vi "S2C_OM8257_Proc_Commands.vi"(7 "VI_Ref":refnum<vi>, 8 "Error In":errorcluster, 10 "Settings":T1, 11 "Q-Ref":refnum<queue>) -> (0 "Error Out":errorcluster, 2 "Stop?":bool, 3 "Response":variant)   [LabVIEW 2015]
uses:
  S2C_OM8257_Proc_Globals.vi
  _Shared/S2C_Shared_Proc_Globals.vi
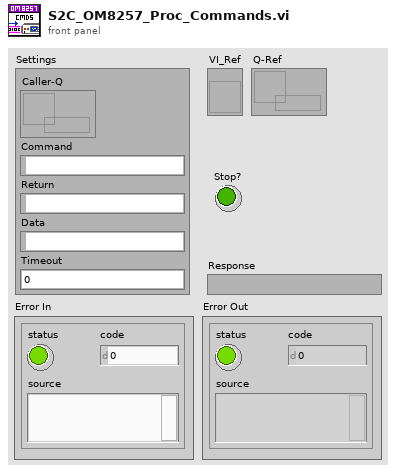
[diagram p1: front panel]
types:
  T1 = cluster{"Caller-Q":refnum<queue>, "Command":string, "Return":string, "Data":variant, "Timeout":dbl}
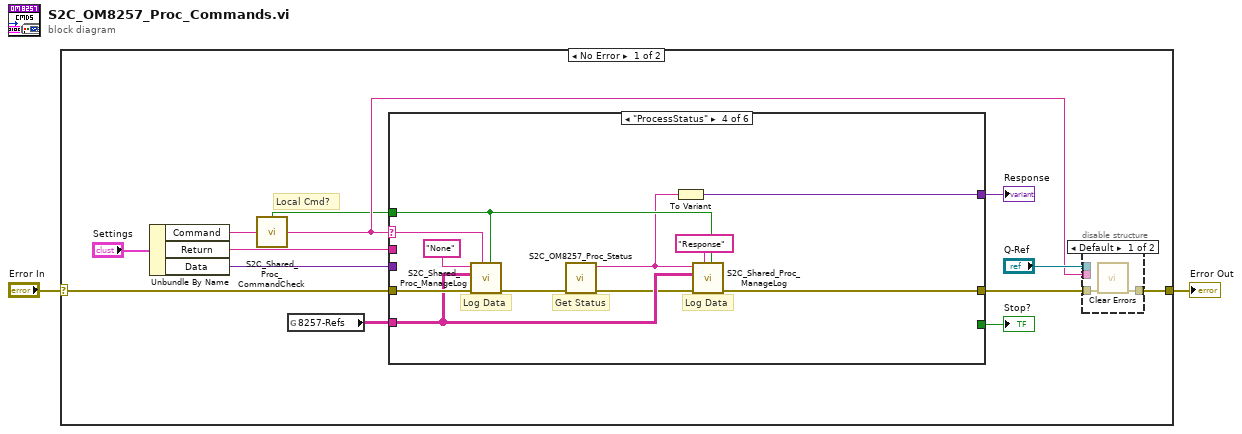
[diagram p0: block diagram]
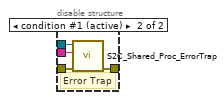
[diagram p2: hidden frame]
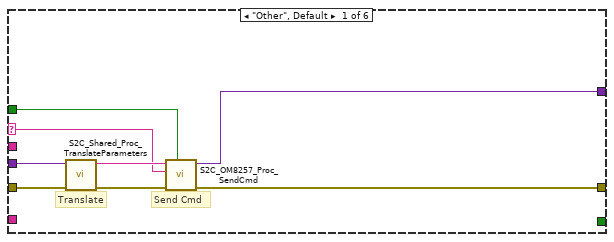
[diagram p3: hidden frame]
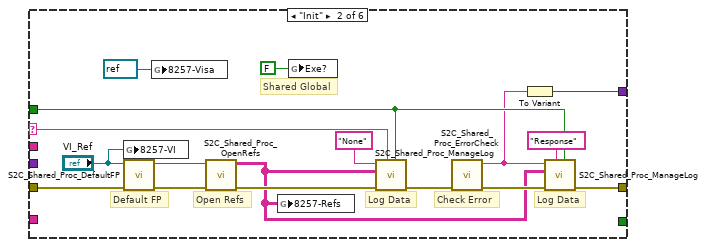
[diagram p4: hidden frame]
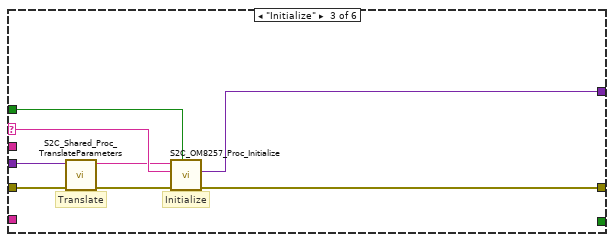
[diagram p5: hidden frame]
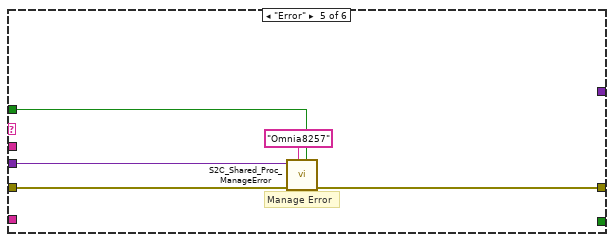
[diagram p6: hidden frame]
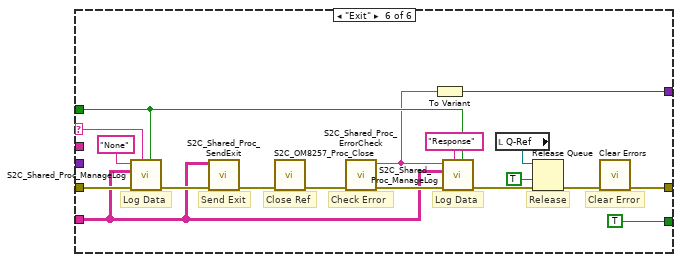
[diagram p7: hidden frame]
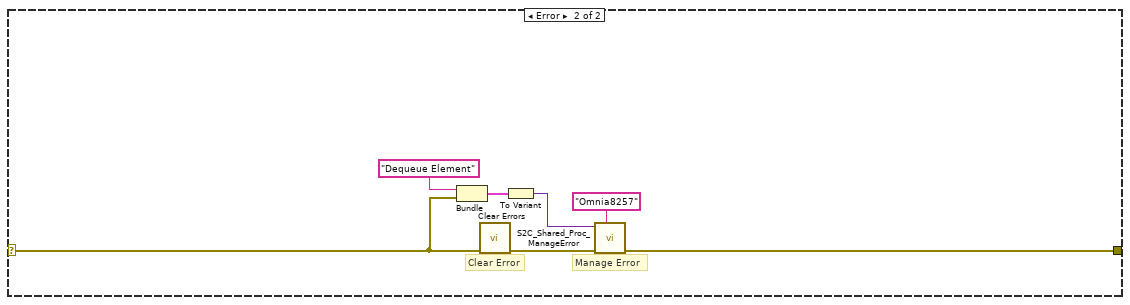
[diagram p8: hidden frame]
diagram:
  n1 = case shown="No Error" "Error In" {
    selector: "Error In" -> [w14 w90]
    tunnel: [w7 w89] -> w1
    frame No Error {
      # "Local Cmd?"
      n2 = Unbundle By Name("Settings") -> ("Command"=w5:string, "Return"=w10:string, "Data"=w15:variant)
      n3 = call "S2C_Shared_Proc_CommandCheck.vi"("Cmd In"=w5) -> ("Local?"=w3:bool, "Cmd Out"=w4:string)  [unwired: 13 in]
      n4 = global read "S2C_OM8257_Proc_Globals.vi" "8257-Refs"() -> (w9:string[][])
      n5 = case shown="\"ProcessStatus\"" w4 {
        selector: w4 -> [w25 w43 w50 w64 _ w85]
        tunnel: w14 -> [w29 w35 w54 w63 w70 w86]
        tunnel: w15 -> [w28 _ w53 _ w68 _]
        tunnel: [w23 w46 w52 w59 w69 w71] -> w8
        tunnel: [w22 w40 w51 w60 _ w79] -> w12
        tunnel: [_ _ _ _ _ TRUE] -> w11
        tunnel: w10 -> [_ _ _ _ _ _]
        tunnel: w3 -> [w24 w44 w47 w62 w66 w83]
        tunnel: w9 -> [_ _ _ w58 _ w76]
        frame "Other", Default {
          # "Send Cmd"
          # "Translate"
          n6 = call "S2C_Shared_Proc_TranslateParameters.vi"("Error In"=w29, "Data"=w28) -> ("Error Out"=w27:errorcluster, "JSON Cluster"=w26:string)  [unwired: 8 in]
          n7 = call "S2C_OM8257_Proc_SendCmd.vi"("Local?"=w24, "Error In"=w27, "Command"=w25, "JSON String"=w26) -> ("Error Out"=w23:errorcluster, "Response"=w22:variant)  [unwired: 6 in]
        }
        frame "Init" {
          # "Default FP"
          # "Shared Global"
          # "Check Error"
          # "Log Data"
          # "Open Refs"
          # "Log Data"
          n8 = global write "S2C_OM8257_Proc_Globals.vi" "8257-VI"("VI_Ref") -> ()
          n9 = call "S2C_Shared_Proc_DefaultFP.vi"("Error In"=w35, "VI_Ref In"="VI_Ref") -> ("Error Out"=w33:errorcluster, "VI_Ref Out"=w34:refnum<vi>)  [unwired: 8 in]
          n10 = global write "S2C_OM8257_Proc_Globals.vi" "8257-Visa"(refnum<visa-resource-name> refnum ("SerialRef")) -> ()
          n11 = call "S2C_Shared_Proc_OpenRefs.vi"("Error In"=w33, "VI_Ref"=w34) -> ("Error Out"=w36:errorcluster, "Refs"=w31:string[][])  [unwired: 8 in]
          n12 = global write "S2C_OM8257_Proc_Globals.vi" "8257-Refs"(w31) -> ()
          n13 = global write "S2C_Shared_Proc_Globals.vi" "Exe?"(FALSE ("Exe?")) -> ()
          n14 = call "S2C_Shared_Proc_ManageLog.vi"("Local?"=w44, "Command"=w43, "Error In"=w36, "Refs"=w31, "Data In"="None") -> ("Error Out"=w38:errorcluster)  [unwired: 5 in, 1 out]
          n15 = call "S2C_Shared_Proc_ErrorCheck.vi"("Error In"=w38) -> ("Error Out"=w41:errorcluster, "Status"=w39:string)  [unwired: 9 in]
          n16 = To Variant(anything=w39) -> (Variant=w40:variant)
          n17 = call "S2C_Shared_Proc_ManageLog.vi"("Local?"=w44, "Command"="Response", "Error In"=w41, "Refs"=w31, "Data In"=w39) -> ("Error Out"=w46:errorcluster)  [unwired: 5 in, 1 out]
        }
        frame "Initialize" {
          # "Initialize"
          # "Translate"
          n18 = call "S2C_Shared_Proc_TranslateParameters.vi"("Error In"=w54, "Data"=w53) -> ("Error Out"=w49:errorcluster, "JSON Cluster"=w48:string)  [unwired: 8 in]
          n19 = call "S2C_OM8257_Proc_Initialize.vi"("Local?"=w47, "Error In"=w49, "Command"=w50, "JSON String"=w48) -> ("Error Out"=w52:errorcluster, "Response"=w51:variant)  [unwired: 6 in]
        }
        frame "ProcessStatus" {
          # "Get Status"
          # "Log Data"
          # "Log Data"
          n20 = call "S2C_Shared_Proc_ManageLog.vi"("Local?"=w62, "Command"=w64, "Error In"=w63, "Refs"=w58, "Data In"="None") -> ("Error Out"=w57:errorcluster)  [unwired: 5 in, 1 out]
          n21 = call "S2C_OM8257_Proc_Status.vi"("Error In"=w57) -> ("Error Out"=w56:errorcluster, "Response"=w55:string)  [unwired: 9 in]
          n22 = To Variant(anything=w55) -> (Variant=w60:variant)
          n23 = call "S2C_Shared_Proc_ManageLog.vi"("Local?"=w62, "Command"="Response", "Error In"=w56, "Refs"=w58, "Data In"=w55) -> ("Error Out"=w59:errorcluster)  [unwired: 5 in, 1 out]
        }
        frame "Error" {
          # "Manage Error"
          n24 = call "S2C_Shared_Proc_ManageError.vi"("Local?"=w66, "Process"="Omnia8257", "Error In"=w70, "Data"=w68) -> ("Error Out"=w69:errorcluster)  [unwired: 7 in]
        }
        frame "Exit" {
          # "Clear Error"
          # "Release"
          # "Check Error"
          # "Send Exit"
          # "Log Data"
          # "Close Ref"
          # "Log Data"
          n25 = call "S2C_Shared_Proc_ManageLog.vi"("Local?"=w83, "Command"=w85, "Error In"=w86, "Refs"=w76, "Data In"="None") -> ("Error Out"=w77:errorcluster)  [unwired: 5 in, 1 out]
          n26 = call "S2C_Shared_Proc_SendExit.vi"("Error In"=w77, "Refs"=w76) -> ("Error Out"=w75:errorcluster)  [unwired: 9 in]
          n27 = call "S2C_OM8257_Proc_Close.vi"("Error In"=w75) -> ("Error Out"=w84:errorcluster)  [unwired: 10 in]
          n28 = call "S2C_Shared_Proc_ErrorCheck.vi"("Error In"=w84) -> ("Error Out"=w81:errorcluster, "Status"=w78:string)  [unwired: 9 in]
          n29 = To Variant(anything=w78) -> (Variant=w79:variant)
          n30 = call "S2C_Shared_Proc_ManageLog.vi"("Local?"=w83, "Command"="Response", "Error In"=w81, "Refs"=w76, "Data In"=w78) -> ("Error Out"=w80:errorcluster)  [unwired: 5 in, 1 out]
          n31 = local read "Q-Ref"() -> (w73:refnum<queue>)
          n32 = Release Queue(queue=w73, force destroy? (F)=TRUE, error in (no error)=w80) -> (error out=w74:errorcluster)  [unwired: 2 out]
          n33 = call <vilib>:"Clear Errors.vi"("error in (no error)"=w74) -> ("error out"=w71:errorcluster)  [unwired: 5 in, 1 out]
        }
      }
      "Response" <- w12
      "Stop?" <- w11
      n34 = disable-structure shown="Default" {
        disable-tunnel: w8 -> [w17 w21]
        disable-tunnel: [w16 w20] -> w7
        disable-tunnel: w4 -> [_ w19]
        disable-tunnel: "Q-Ref" -> [_ w18]
        frame condition #0 {
          n35 = call <vilib>:"Clear Errors.vi"("error in (no error)"=w17) -> ("error out"=w16:errorcluster)  [unwired: 5 in, 1 out]
        }
        frame condition #1 (active) {
          # "Error Trap"
          n36 = call "S2C_Shared_Proc_ErrorTrap.vi"("Error In"=w21, "Command"=w19, "Q-Ref"=w18) -> ("Error Out"=w20:errorcluster)  [unwired: 8 in]
        }
      }
    }
    frame Error {
      # "Clear Error"
      # "Manage Error"
      n37 = Bundle("Dequeue Element", "error IO"=w90) -> (w94:cluster{string, "error IO":errorcluster})  [unwired: 1 in]
      n38 = call <vilib>:"Clear Errors.vi"("error in (no error)"=w90) -> ("error out"=w91:errorcluster)  [unwired: 5 in, 1 out]
      n39 = To Variant(anything=w94) -> (Variant=w92:variant)
      n40 = call "S2C_Shared_Proc_ManageError.vi"("Process"="Omnia8257", "Error In"=w91, "Data"=w92) -> ("Error Out"=w89:errorcluster)  [unwired: 8 in]
    }
  }
  "Error Out" <- w1
